vi "build_boolian_array.vi"(8 "error in (no error)":errorcluster, 11 "card":u16(ring) items=["card 1", "card 2"]) -> (0 "error out":errorcluster)   [LabVIEW 2018]
doc: "builds a boolian array from the current state of the switches card 1 (V1-V8) or card 2 (V9-V11)"
panel:
  in  "vi reference":refnum<vi>
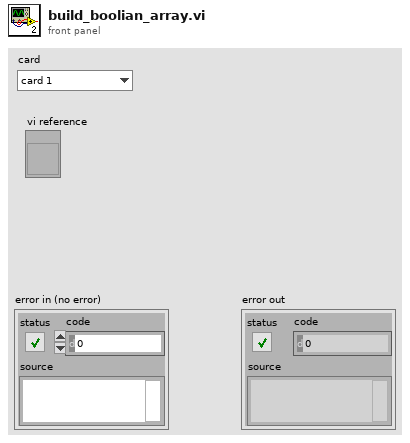
[diagram p1: front panel]
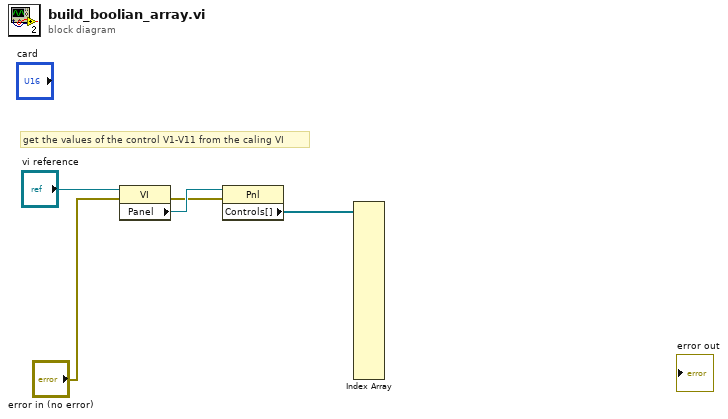
[diagram p0: block diagram]
diagram:
  # "get the values of the control V1-V11 from the caling VI"
  n1 = property class="VI"(reference="vi reference", error in="error in (no error)") -> (error out=w2:errorcluster, "Panel"=w4:refnum<vi>)  [unwired: 1 out]
  n2 = property class="Pnl"(reference=w4, error in=w2) -> ("Controls[]"=w1:refnum<vi>[])  [unwired: 2 out]
  n3 = Index Array(array=w1) -> ()  [unwired: 20 in, 20 out]
